vi "Item count.vi"(11 "MsgPackMap in":refnum<class "MsgPackMap.lvclass">) -> (2 "Count":i32, 3 "MsgPackMap out":refnum<class "MsgPackMap.lvclass">)   [LabVIEW 2020, in "MessagePack.lvlib" / "MsgPackMap.lvclass"]
uses:
  MsgPackMap.lvclass
  MsgPackMap.lvclass/MsgPackMap.ctl
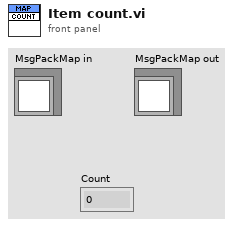
[diagram p1: front panel]
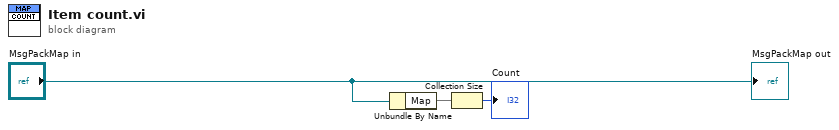
[diagram p0: block diagram]
diagram:
  n1 = Unbundle By Name("MsgPackMap in") -> ("Map"=w2:map{u8[], u8[]})
  n2 = Collection Size(1:w2) -> (0:→"Count":i32)
  "MsgPackMap out" <- "MsgPackMap in"
